vi "NI 9237 Getting Started (FPGA).vi"() -> ()   [LabVIEW 2019]
uses:
  <vilib>/eio/EIONode/EIONode.xnode
  <vilib>/eio/EIOPropertyNode/EIOPropertyNode.xnode
  <vilib>/rvi/DataTransferAndStorage/Container/XNode/niFpgaContainer.xnode
  <vilib>/rvi/eio/common/nirviEmuTemplatePropertyGet_errors.vi
  <vilib>/rvi/eio/common/nirviEmuTemplatePropertyGet_noerrors.vi
  <vilib>/rvi/eio/common/nirviEmuTemplatePropertySet_errors.vi
  <vilib>/rvi/eio/common/nirviEmuTemplatePropertySet_noerrors.vi
  <vilib>/rvi/eio/common/nirviEmuTemplateMethod_errors.vi
  <vilib>/LabVIEW Targets/FPGA/cRIO/shared/nicrio_ModuleControls/nicrio_cRIO-9237_DataRatesRing.ctl
  <vilib>/LabVIEW Targets/FPGA/cRIO/shared/nicrio_ModuleControls/nicrio_cRIO-9237_ExcitationVoltageRing.ctl
  <vilib>/rvi/interface/RandomDataEmulation/nirviRandomDataFpgaReadWriteTemplate.vi
panel:
  in  "Half-Bridge Enable":bool
  in  "Excitation Voltage":T1 items=["2.5 Volts", "3.3 Volts", "5.0 Volts", "10.0 Volts", "External Excitation"]
  in  "Finite?":bool=TRUE
  in  "Stop Button":bool
  out "FIFO Full":bool
  in  "Data Rate":T2=1 items=["50.000 kS/s (NI 9237)"=1, "25.000 kS/s (NI 9237)"=2, "16.667 kS/s (NI 9237)"=3, "12.500 kS/s (NI 9237)"=4, "10.000 kS/s (NI 9237)"=5, "8.333 kS/s (NI 9237)"=6, "7.143 kS/s (NI 9237)"=7, "6.250 kS/s (NI 9237)"=8, "5.556 kS/s (NI 9237)"=9, "5.000 kS/s (NI 9237)"=10, "4.545 kS/s (NI 9237)"=11, "4.167 kS/s (NI 9237)"=12, "3.846 kS/s (NI 9237)"=13, "3.571 kS/s (NI 9237)"=14, "3.333 kS/s (NI 9237)"=15, "3.125 kS/s (NI 9237)"=16, "2.941 kS/s (NI 9237)"=17, "2.778 kS/s (NI 9237)"=18, "2.632 kS/s (NI 9237)"=19, "2.500 kS/s (NI 9237)"=20, "2.381 kS/s (NI 9237)"=21, "2.273 kS/s (NI 9237)"=22, "2.174 kS/s (NI 9237)"=23, "2.083 kS/s (NI 9237)"=24, "2.000 kS/s (NI 9237)"=25, "1.923 kS/s (NI 9237)"=26, "1.852 kS/s (NI 9237)"=27, "1.786 kS/s (NI 9237)"=28, "1.724 kS/s (NI 9237)"=29, "1.667 kS/s (NI 9237)"=30, "1.613 kS/s (NI 9237)"=31]
  in  "Shunt Cal Enable":bool
  in  "Samples per Channel":u32=1000
  out "error out":errorcluster {"code" format="%.0x"}
  # "Overview: Demonstrates how to acquire and scale the data from the NI 9237. \nRequirements: LabVIEW Full Development System, LV FPGA, and NI RIO\nInstructions: \n1. Run NI 9237 Getting Started (Host).vi"
  # "Timing Parameters"
  # "Output Parameters"
  # "Input Parameters"
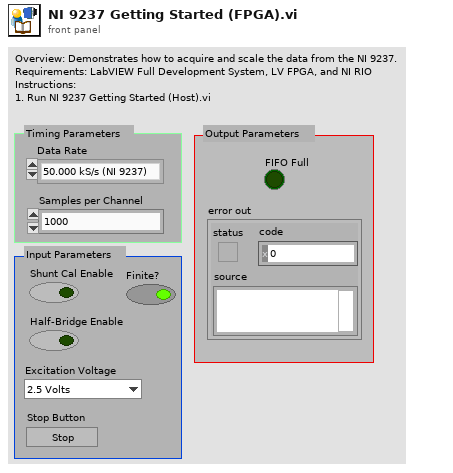
[diagram p1: front panel]
types:
  T1 = typedef "nicrio_cRIO-9237_ExcitationVoltageRing.ctl" = u8
  T2 = typedef "nicrio_cRIO-9237_DataRatesRing.ctl" = u8
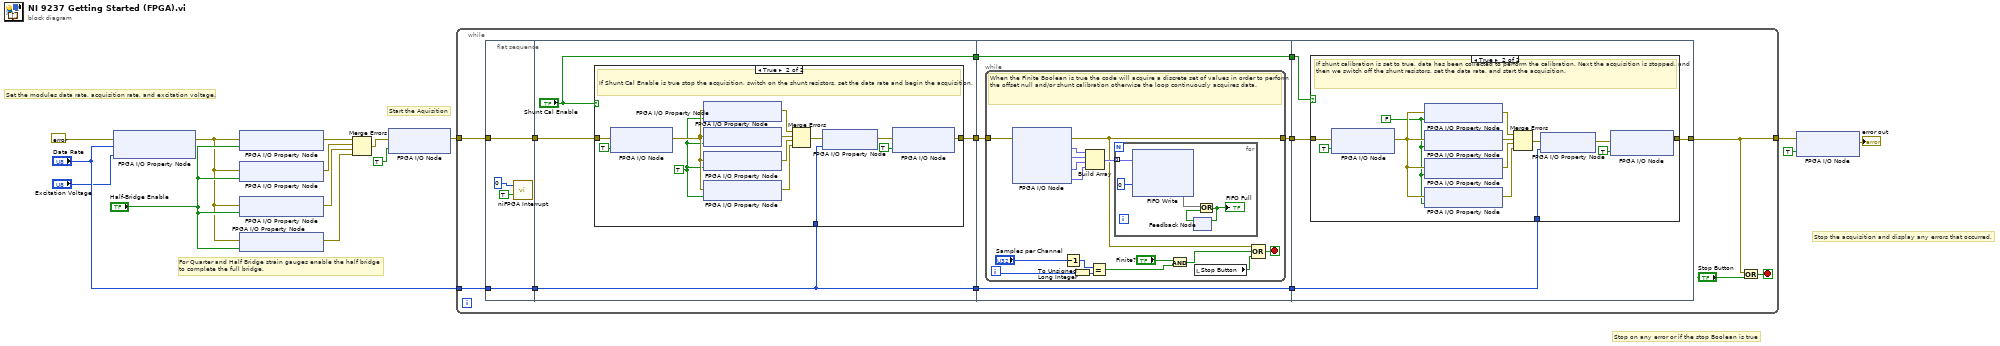
[diagram p0: block diagram]
diagram:
  # "Stop the acquisition and display any errors that occurred."
  # "Stop on any error or if the stop Boolean is true"
  # "Start the Aquisition"
  # "For Quarter and Half Bridge strain gauges enable the half bridge \nto complete the full bridge."
  # "Set the modules data rate, acquisition rate, and excitation voltage."
  n1 = xnode "FPGA I/O Property Node"("error in"=errorcluster {"status"=FALSE, "code"=0, "source"=""}, "Data Rate"="Data Rate", "Excitation Voltage"="Excitation Voltage") -> ("error out"=w2:errorcluster)  [unwired: 1 in, 1 out]
  n2 = xnode "FPGA I/O Property Node"("error in"=w2, "Half-Bridge Enable"="Half-Bridge Enable") -> ("error out"=w6:errorcluster)  [unwired: 1 in, 1 out]
  n3 = xnode "FPGA I/O Property Node"("error in"=w2, "Half-Bridge Enable"="Half-Bridge Enable") -> ("error out"=w5:errorcluster)  [unwired: 1 in, 1 out]
  n4 = xnode "FPGA I/O Property Node"("error in"=w2, "Half-Bridge Enable"="Half-Bridge Enable") -> ("error out"=w4:errorcluster)  [unwired: 1 in, 1 out]
  n5 = xnode "FPGA I/O Property Node"("error in"=w2, "Half-Bridge Enable"="Half-Bridge Enable") -> ("error out"=w3:errorcluster)  [unwired: 1 in, 1 out]
  n6 = Merge Errors(w6, w5, w4, w3) -> (w1:errorcluster)
  n7 = xnode "FPGA I/O Node"("error in"=w1, "Mod1/Start"=TRUE ("Mod1/Stop")) -> ("error out"=w13:errorcluster)  [unwired: 1 in, 1 out]
  n8 = while {
    tunnel: w13 -> [w28]
    tunnel: [w25] -> w11
    tunnel: "Data Rate" -> [w20]
    stop <- w26 stop-if-true
    n9 = flat-sequence {
      tunnel: w28 -> [w32]
      tunnel: [w32] -> w23
      tunnel: [w29] -> w21
      tunnel: w20 -> [w29]
      tunnel: w23 -> [w36]
      tunnel: [w35] -> w22
      tunnel: w21 -> [w34]
      tunnel: [w34] -> w18
      tunnel: ["Shunt Cal Enable"] -> w17
      tunnel: [w53] -> w27
      tunnel: w22 -> [w54]
      tunnel: [w52] -> w19
      tunnel: w18 -> [w52]
      tunnel: w17 -> [w51]
      tunnel: [w51] -> w16
      tunnel: [w78] -> w25
      tunnel: w27 -> [w79]
      tunnel: w19 -> [w76]
      tunnel: w16 -> [w77]
      frame #0 {
        n10 = call <vilib>:"niFPGA Interrupt.vi"("Wait Until Cleared (F)"=TRUE, "IRQ Number (0)"=u8 0) -> ()  [unwired: 1 in]
      }
      frame #1 {
        n11 = case shown="True" "Shunt Cal Enable" {
          tunnel: w36 -> [w37 w47]
          tunnel: [w37 w45] -> w35
          tunnel: w34 -> [_ w42]
          frame False {
          }
          frame True {
            w40 = TRUE ("Shunt Cal Enable")
            # "If Shunt Cal Enable is true stop the acquisition, switch on the shunt resistors, set the data rate and begin the acquisition."
            n12 = xnode "FPGA I/O Node"("error in"=w47, "Mod1/Stop"=TRUE) -> ("error out"=w46:errorcluster)  [unwired: 1 in, 1 out]
            n13 = xnode "FPGA I/O Property Node"("error in"=w46, "Shunt Cal Enable"=w40) -> ("error out"=w50:errorcluster)  [unwired: 1 in, 1 out]
            n14 = xnode "FPGA I/O Property Node"("error in"=w46, "Shunt Cal Enable"=w40) -> ("error out"=w38:errorcluster)  [unwired: 1 in, 1 out]
            n15 = xnode "FPGA I/O Property Node"("error in"=w46, "Shunt Cal Enable"=w40) -> ("error out"=w49:errorcluster)  [unwired: 1 in, 1 out]
            n16 = xnode "FPGA I/O Property Node"("error in"=w46, "Shunt Cal Enable"=w40) -> ("error out"=w48:errorcluster)  [unwired: 1 in, 1 out]
            n17 = Merge Errors(w50, w38, w49, w48) -> (w43:errorcluster)
            n18 = xnode "FPGA I/O Property Node"("error in"=w43, "Data Rate"=w42) -> ("error out"=w44:errorcluster)  [unwired: 1 in, 1 out]
            n19 = xnode "FPGA I/O Node"("error in"=w44, "Mod1/Start"=TRUE) -> ("error out"=w45:errorcluster)  [unwired: 1 in, 1 out]
          }
        }
      }
      frame #2 {
        n20 = while {
          tunnel: w54 -> [w55]
          tunnel: [w59] -> w53
          i -> [w63]
          stop <- w56 stop-if-true
          # "When the Finite Boolean is true the code will acquire a discrete set of values in order to perform the offset null and/or shunt calibration otherwise the loop continuously acquires data."
          n21 = xnode "FPGA I/O Node"("error in"=w55) -> ("error out"=w59:errorcluster, "Mod1/AI0"=w69:fxp<+/-,24,-4>, "Mod1/AI1"=w68:fxp<+/-,24,-4>, "Mod1/AI2"=w66:fxp<+/-,24,-4>, "Mod1/AI3"=w67:fxp<+/-,24,-4>)  [unwired: 4 in, 4 out]
          n22 = Decrement(x="Samples per Channel") -> (x-1=w65:u32)
          n23 = To Unsigned Long Integer(number=w63) -> (unsigned 32bit integer=w64:u32)
          n24 = Build Array(w69, w68, w66, w67) -> (w70:fxp<+/-,24,-4>[])
          n25 = Equal?(x=w65, y=w64) -> (x = y?=w60:bool)
          n26 = for {
            tunnel: w70 -> [w74] mode=indexing
            n27 = xnode ("FIFO Write")("Element"=w74, "Timeout"=0) -> ("Timed Out?"=w73)  [unwired: 1 in, 1 out]
            n28 = feedback #1() -> (w71:bool)  [unwired: 1 in]
            n29 = Or(x=w73, y=w71) -> (x .or. y?=w72:bool)
            "FIFO Full" <- w72
            n30 = feedback-in #1(w72) -> ()
          }
          n31 = And(x="Finite?", y=w60) -> (x .and. y?=w58:bool)
          n32 = local read "Stop Button"() -> (w57:bool)
          n33 = Compound Arithmetic op=OR(w59, w58, w57) -> (w56:bool)
        }
      }
      frame #3 {
        n34 = case shown="True" w77 {
          tunnel: w79 -> [w80 w89]
          tunnel: [w80 w87] -> w78
          tunnel: w76 -> [_ w84]
          frame False {
          }
          frame True {
            w83 = FALSE ("Shunt Cal Enable")
            # "If shunt calibration is set to true, data has been collected to perform the calibration. Next the acquisition is stopped, and then we switch off the shunt resistors, set the data rate, and start the acquisition."
            n35 = xnode "FPGA I/O Node"("error in"=w89, "Mod1/Stop"=TRUE) -> ("error out"=w88:errorcluster)  [unwired: 1 in, 1 out]
            n36 = xnode "FPGA I/O Property Node"("error in"=w88, "Shunt Cal Enable"=w83) -> ("error out"=w93:errorcluster)  [unwired: 1 in, 1 out]
            n37 = xnode "FPGA I/O Property Node"("error in"=w88, "Shunt Cal Enable"=w83) -> ("error out"=w92:errorcluster)  [unwired: 1 in, 1 out]
            n38 = xnode "FPGA I/O Property Node"("error in"=w88, "Shunt Cal Enable"=w83) -> ("error out"=w91:errorcluster)  [unwired: 1 in, 1 out]
            n39 = xnode "FPGA I/O Property Node"("error in"=w88, "Shunt Cal Enable"=w83) -> ("error out"=w90:errorcluster)  [unwired: 1 in, 1 out]
            n40 = Merge Errors(w93, w92, w91, w90) -> (w85:errorcluster)
            n41 = xnode "FPGA I/O Property Node"("error in"=w85, "Data Rate"=w84) -> ("error out"=w86:errorcluster)  [unwired: 1 in, 1 out]
            n42 = xnode "FPGA I/O Node"("error in"=w86, "Mod1/Start"=TRUE) -> ("error out"=w87:errorcluster)  [unwired: 1 in, 1 out]
          }
        }
      }
    }
    n43 = Or(x=w25, y="Stop Button") -> (x .or. y?=w26:bool)
  }
  n44 = xnode "FPGA I/O Node"("error in"=w11, "Mod1/Stop"=TRUE) -> ("error out"=→"error out":errorcluster)  [unwired: 1 in, 1 out]
